vi "Buttons_test.vi"() -> (0 "Buttons[6]":bool, 2 "OUT":dbl)   [LabVIEW 2020]
uses:
  <vilib>/Rock Robotics/WPI/Utilities/WPI_GetSetVariantRefNum.vi
panel:
  out "Buttons 5":bool
  out "Buttons 4":bool
  out "Multiplicação":dbl
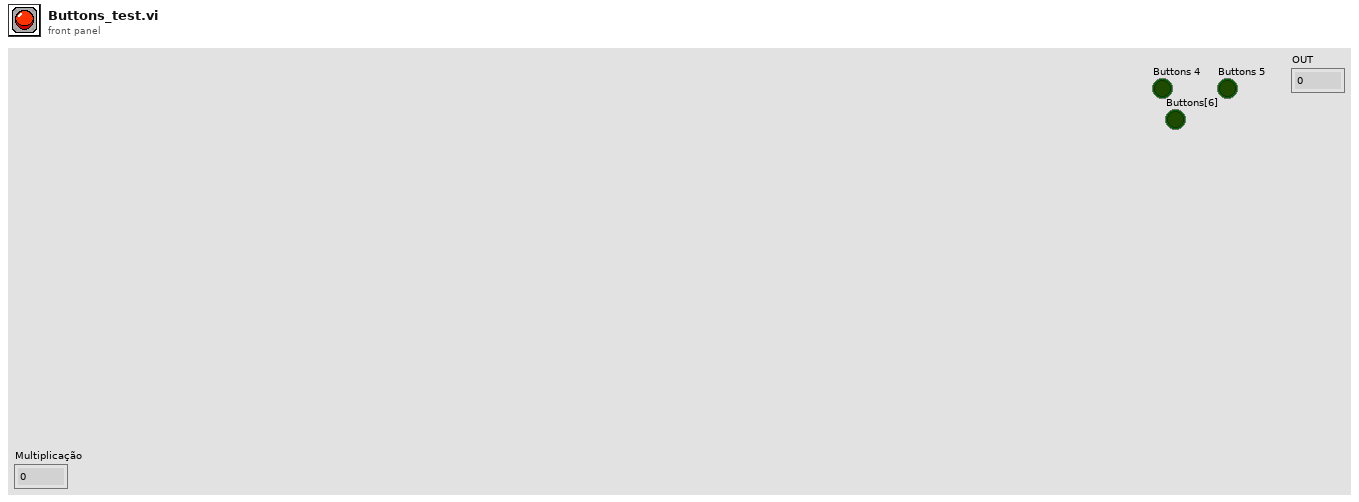
[diagram p1: front panel]
types:
  T1 = typedef "WPI_JoystickDevRef.ctl" = cluster{"Device":T2}
  T2 = typedef "WPI_JoystickDeviceEnum.ctl" = enum16{"USB 0", "USB 1", "USB 2", "USB 3", "USB 4", "USB 5"}
  T3 = cluster{"Buttons[0]":bool, "Buttons[1]":bool, "Buttons[2]":bool, "Buttons[3]":bool, "Buttons[4]":bool, "Buttons[5]":bool, "Buttons[6]":bool, "Buttons[7]":bool, "Buttons[8]":bool}
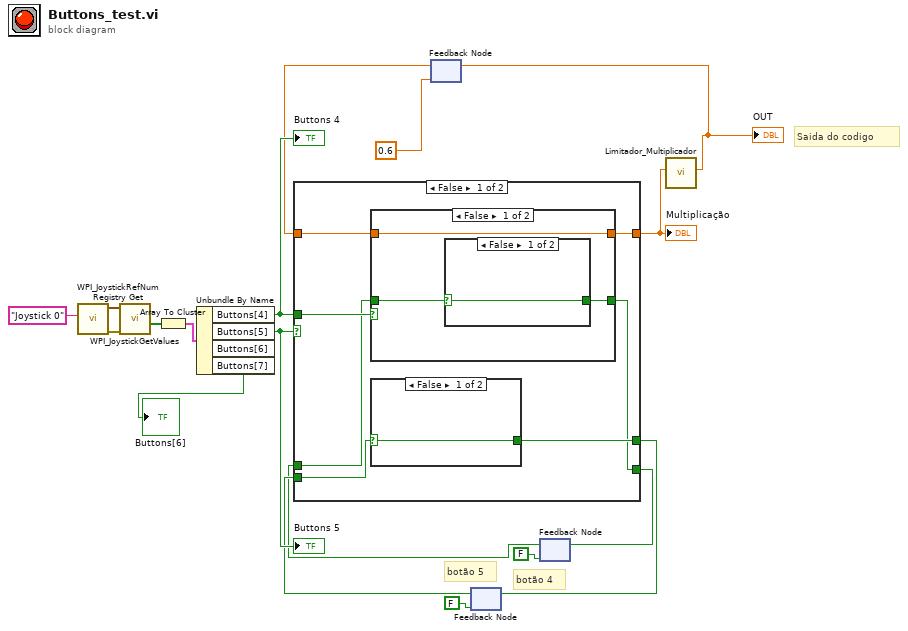
[diagram p0: block diagram]
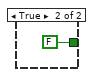
[diagram p2: hidden frame]
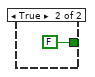
[diagram p3: hidden frame]
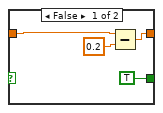
[diagram p5: hidden frame]
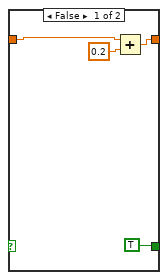
[diagram p7: hidden frame]
diagram:
  # "Saida do codigo"
  # "botão 5"
  # "botão 4"
  n1 = call <vilib>:"WPI_JoystickRefNum Registry Get.vi"("refnum name"="Joystick 0") -> ("error out"=w8:errorcluster, "JoystickDevRef"=w7:T1)  [unwired: 1 in, 8 out]
  n2 = call <vilib>:"WPI_JoystickGetValues.vi"("error in (no error)"=w8, "JoystickDevRef"=w7) -> ("Buttons"=w5:bool[])  [unwired: 5 in, 4 out]
  n3 = Array To Cluster(array=w5) -> (cluster=w18:T3)
  n4 = Unbundle By Name(w18) -> ("Buttons[4]"=w17:bool, "Buttons[5]"=w16:bool, "Buttons[7]"=→"Buttons[6]":bool)  [unwired: 1 out]
  "Buttons 4" <- w17
  "Buttons 5" <- w16
  n5 = feedback #1(0.6 ("y")) -> (w2:dbl)
  n6 = feedback #2(FALSE) -> (w13:bool)
  n7 = feedback #3(FALSE) -> (w11:bool)
  n8 = case shown="False" w16 {
    tunnel: w17 -> [w25 _]
    tunnel: [w23 w45] -> w9
    tunnel: w2 -> [w24 w46]
    tunnel: w13 -> [w22 w47]
    tunnel: [w21 w44] -> w12
    tunnel: w11 -> [w20 w43]
    tunnel: [w19 w43] -> w10
    frame False {
      n9 = case shown="False" w25 {
        tunnel: w24 -> [w30 w36]
        tunnel: [w30 w35] -> w23
        tunnel: w20 -> [w29 w34]
        tunnel: [w28 w33] -> w19
        frame False {
          n10 = case shown="False" w29 {
            selector: w29 -> [w31 _]
            tunnel: [w31 FALSE] -> w28
            frame False {
            }
            frame True {
            }
          }
        }
        frame True {
          n11 = case shown="True" w34 {
            selector: w34 -> [_ w41]
            tunnel: w36 -> [w39 w42]
            tunnel: [w38 w42] -> w35
            tunnel: [TRUE w41] -> w33
            frame False {
              n12 = Subtract(x=w39, y=0.2) -> (x-y=w38:dbl)
            }
            frame True {
            }
          }
        }
      }
      n13 = case shown="False" w22 {
        selector: w22 -> [w26 _]
        tunnel: [w26 FALSE] -> w21
        frame False {
        }
        frame True {
        }
      }
    }
    frame True {
      n14 = case shown="True" w47 {
        selector: w47 -> [_ w52]
        tunnel: w46 -> [w50 w53]
        tunnel: [w49 w53] -> w45
        tunnel: [TRUE w52] -> w44
        frame False {
          n15 = Add(x=w50, y=0.2) -> (x+y=w49:dbl)
        }
        frame True {
        }
      }
    }
  }
  "Multiplicação" <- w9
  n16 = feedback-in #2(w12) -> ()
  n17 = feedback-in #3(w10) -> ()
  n18 = call "Limitador_Multiplicador.vi"("IN"=w9) -> ("OUT"=w4:dbl)  [unwired: 10 in]
  "OUT" <- w4
  n19 = feedback-in #1(w4) -> ()
